vi "LEBITplc.Bob1toBunMonitor.vi"(0 "i ref in":refnum<vi>, 1 "data":i8[](array[numeric]), 2 "i attribute in":T1, 3 "index":i32, 4 "NickNames":string, 5 "error in":errorcluster, 7 "no link":bool) -> (14 "i ref out":refnum<vi>, 15 "Data":dbl[](array[numeric]), 16 "i attribute out":T1, 17 "Indexs":i32[](array[numeric]), 19 "error out":errorcluster)   [LabVIEW 2014, in "LEBITplc.lvlib"]
uses:
  LEBITplc.lvlib
  LEBITplc.i attribute.ctl
panel:
  out "No Link":bool
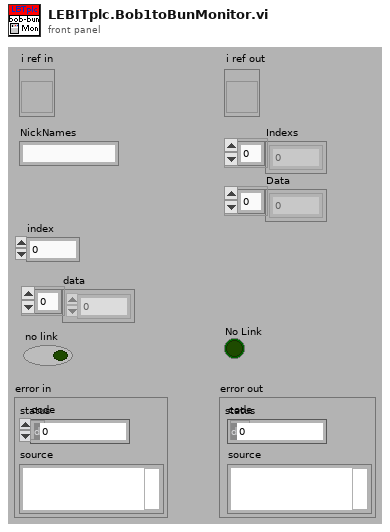
[diagram p1: front panel]
types:
  T1 = typedef "LEBITplc.lvlib/LEBITplc.i attribute.ctl" = cluster{"LLFLocation":string, "SetFileLocation":string, "nickNames":string[], "setValuePLCServiceID":i32[], "GUIServiceID":i32[], "monValuePLC":string[], "SetValueServiceID":i32[], "MonValueServiceID":i32[], "SetValue":dbl[][], "SetValueMin":dbl[], "SetValueMax":dbl[], "SetValueInfoServiceID":i32[], "GUINames":string[], "ListOfBases":string[], "Scale":dbl[], "Offset":dbl[], "setValuePLC":string[], "BaseName":string[], "ScaleServiceID":i32[], "OffsetServiceID":i32[], "AllPLCValues":string[], "CondSpecialArray":string[][], "CondSpecialIndex":i32[], "CondSpecialMonValue":dbl[], "RecentlyChanged":i32[], "SetFileLocationID":i32, "Dependent-Monitors":string[][], "LastLoadedFiles":string[], "IonGuideCalibLocation":string, "Monitor Dependent":string[], "Special":string[], "PLC?":bool[], "Start Date":string, "ListOfBasesServiceID":i32, "SETRA VISA resource":refnum<visa-resource-name>}
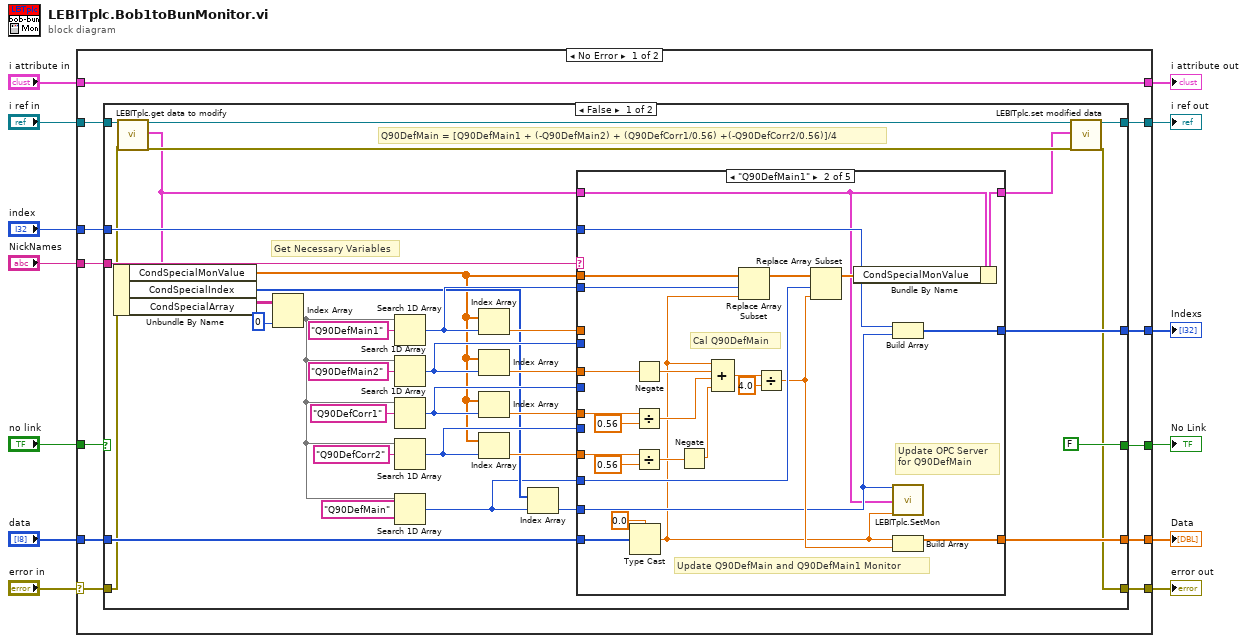
[diagram p0: block diagram]
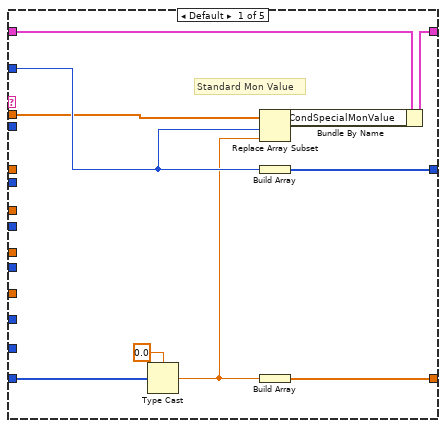
[diagram p2: hidden frame]
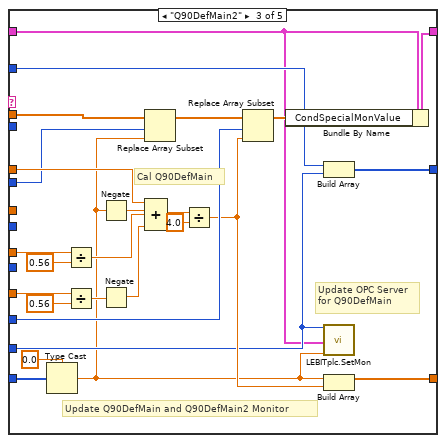
[diagram p3: hidden frame]
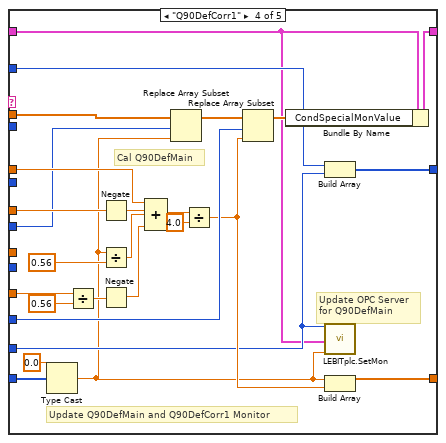
[diagram p4: hidden frame]
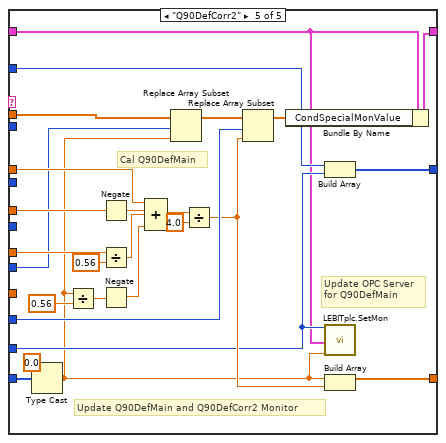
[diagram p5: hidden frame]
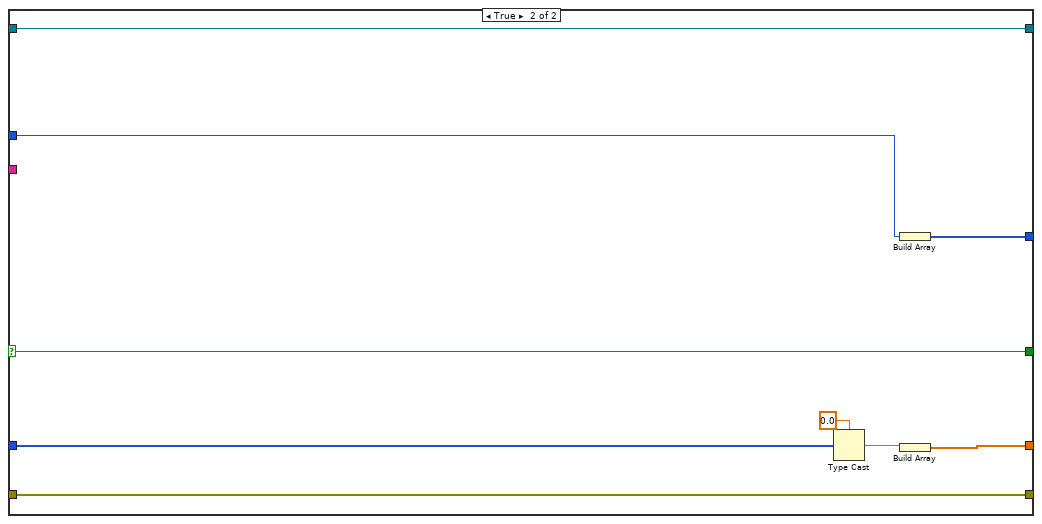
[diagram p6: hidden frame]
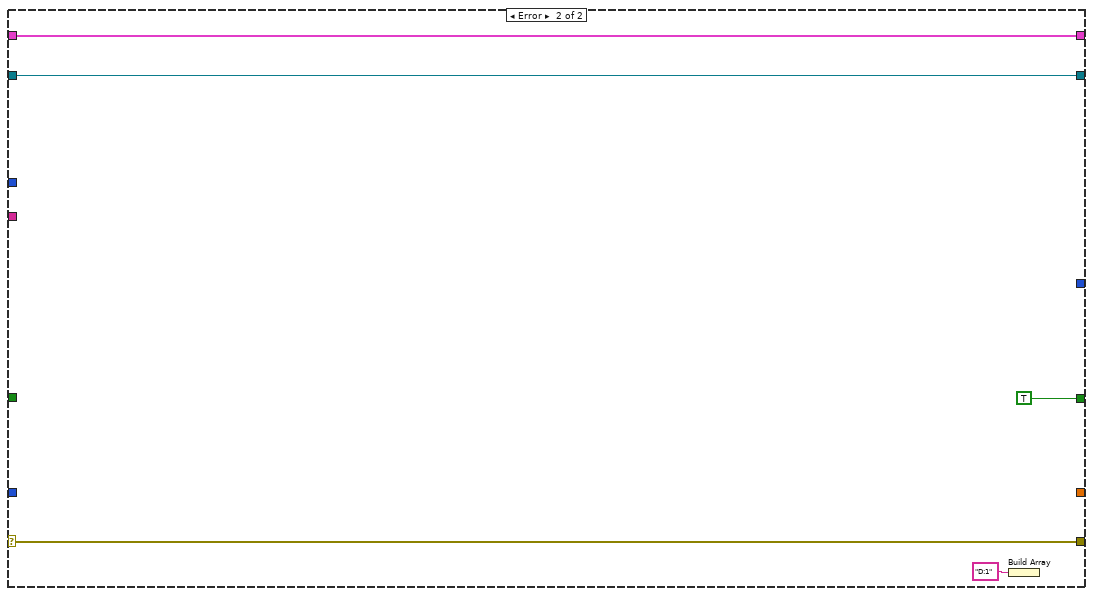
[diagram p7: hidden frame]
diagram:
  n1 = case shown="No Error" "error in" {
    selector: "error in" -> [w19 w187]
    tunnel: "NickNames" -> [w25 _]
    tunnel: [w20 w187] -> w12
    tunnel: "data" -> [w24 _]
    tunnel: "i attribute in" -> [w16 w185]
    tunnel: "i ref in" -> [w21 w186]
    tunnel: [w15 w186] -> w7
    tunnel: "index" -> [w23 _]
    tunnel: [w16 w185] -> w5
    tunnel: [w22 _] -> w4
    tunnel: "no link" -> [w18 _]
    tunnel: [w17 TRUE] -> w2
    tunnel: [w14 _] -> w1
    frame No Error {
      n2 = case shown="False" w18 {
        selector: w18 -> [_ w180]
        tunnel: w25 -> [w55 _]
        tunnel: w24 -> [w54 w175]
        tunnel: w23 -> [w48 w179]
        tunnel: [w47 w178] -> w22
        tunnel: w21 -> [w40 w182]
        tunnel: [w37 w182] -> w15
        tunnel: [w27 w181] -> w20
        tunnel: w19 -> [w26 w181]
        tunnel: [FALSE w180] -> w17
        tunnel: [w30 w174] -> w14
        frame False {
          # "Q90DefMain = [Q90DefMain1 + (-Q90DefMain2) + (Q90DefCorr1/0.56) +(-Q90DefCorr2/0.56)]/4"
          # "Get Necessary Variables"
          n3 = call "LEBITplc.get data to modify.vi"("i ref in"=w40, "error in (no error)"=w26) -> ("i ref out"=w39:refnum<vi>, "i attribute"=w28:T1, "error out"=w38:errorcluster)  [unwired: 14 in, 1 out]
          n4 = Unbundle By Name(w28) -> ("CondSpecialMonValue"=w32:dbl[], "CondSpecialIndex"=w33:i32[], "CondSpecialArray"=w59:string[][])
          n5 = Index Array(array=w59, index (col)=0 ("index (row)")) -> (element=w34:string[])  [unwired: 1 in]
          n6 = Search 1D Array(1D array=w34, element="Q90DefMain1") -> (index of element=w45:i32)  [unwired: 1 in]
          n7 = Search 1D Array(1D array=w34, element="Q90DefMain2") -> (index of element=w43:i32)  [unwired: 1 in]
          n8 = Search 1D Array(1D array=w34, element="Q90DefCorr1") -> (index of element=w44:i32)  [unwired: 1 in]
          n9 = Search 1D Array(1D array=w34, element="Q90DefCorr2") -> (index of element=w42:i32)  [unwired: 1 in]
          n10 = Search 1D Array(1D array=w34, element="Q90DefMain") -> (index of element=w29:i32)  [unwired: 1 in]
          n11 = Index Array(array=w32, index=w45) -> (element=w51:dbl)
          n12 = Index Array(array=w32, index=w43) -> (element=w50:dbl)
          n13 = Index Array(array=w32, index=w44) -> (element=w49:dbl)
          n14 = Index Array(array=w32, index=w42) -> (element=w53:dbl)
          n15 = Index Array(array=w33, index=w29) -> (element=w31:i32)
          n16 = case shown="\"Q90DefMain1\"" w55 {
            tunnel: w54 -> [w63 w94 w120 w146 w172]
            tunnel: w53 -> [_ w85 w112 w139 _]
            tunnel: w51 -> [_ _ w103 w130 w157]
            tunnel: w50 -> [_ w89 _ w128 w155]
            tunnel: w49 -> [_ w88 w115 _ w154]
            tunnel: w48 -> [w66 w78 w106 w133 w160]
            tunnel: [w69 w80 w108 w135 w162] -> w47
            tunnel: w28 -> [w67 w71 w97 w123 w149]
            tunnel: [w68 w91 w117 w143 w169] -> w36
            tunnel: w45 -> [_ w73 _ _ _]
            tunnel: w44 -> [_ _ _ w125 _]
            tunnel: w43 -> [_ _ w99 _ _]
            tunnel: w32 -> [w62 w93 w119 w145 w171]
            tunnel: w42 -> [_ _ _ _ w151]
            tunnel: w31 -> [_ w72 w98 w124 w150]
            tunnel: w29 -> [_ w79 w107 w134 w161]
            tunnel: [w61 w74 w100 w126 w152] -> w30
            frame Default {
              # "Standard Mon Value"
              n17 = Type Cast(type=0.0 ("y"), x=w63) -> (*(type *) &x=w60:dbl)
              n18 = Replace Array Subset(array=w62, new element=w60, index=w66) -> (w65:dbl[])
              n19 = Build Array(w66) -> (w69:i32[])
              n20 = Build Array(w60) -> (w61:dbl[])
              n21 = Bundle By Name(cluster=w67, "CondSpecialMonValue"=w65) -> (w68:T1)
            }
            frame "Q90DefMain1" {
              # "Update Q90DefMain and Q90DefMain1 Monitor"
              # "Update OPC Server\nfor Q90DefMain"
              # "Cal Q90DefMain"
              n22 = Type Cast(type=0.0 ("y"), x=w94) -> (*(type *) &x=w70:dbl)
              n23 = Negate(x=w89) -> (-x=w83:dbl)
              n24 = Divide(x=w88, y=0.56) -> (x/y=w82:dbl)
              n25 = Divide(x=w85, y=0.56) -> (x/y=w84:dbl)
              n26 = Negate(x=w84) -> (-x=w81:dbl)
              n27 = Compound Arithmetic op=ADD(w70, w83, w82, w81) -> (w76:dbl)
              n28 = Replace Array Subset(array=w93, new element=w70, index=w73) -> (w92:dbl[])
              n29 = Divide(x=w76, y=4.0) -> (x/y=w75:dbl)
              n30 = Replace Array Subset(array=w92, new element=w75, index=w79) -> (w90:dbl[])
              n31 = Bundle By Name(cluster=w71, "CondSpecialMonValue"=w90) -> (w91:T1)
              n32 = Build Array(w78, w72) -> (w80:i32[])
              n33 = call "LEBITplc.SetMon.vi"("index of element"=w72, "i attribute in"=w71, "Data"=w70) -> ()  [unwired: 17 in]
              n34 = Build Array(w70, w75) -> (w74:dbl[])
            }
            frame "Q90DefMain2" {
              # "Cal Q90DefMain"
              # "Update OPC Server\nfor Q90DefMain"
              # "Update Q90DefMain and Q90DefMain2 Monitor"
              n35 = Type Cast(type=0.0 ("y"), x=w120) -> (*(type *) &x=w96:dbl)
              n36 = Divide(x=w115, y=0.56) -> (x/y=w110:dbl)
              n37 = Divide(x=w112, y=0.56) -> (x/y=w111:dbl)
              n38 = Negate(x=w96) -> (-x=w102:dbl)
              n39 = Negate(x=w111) -> (-x=w109:dbl)
              n40 = Replace Array Subset(array=w119, new element=w96, index=w99) -> (w118:dbl[])
              n41 = Compound Arithmetic op=ADD(w103, w102, w110, w109) -> (w105:dbl)
              n42 = Divide(x=w105, y=4.0) -> (x/y=w101:dbl)
              n43 = Replace Array Subset(array=w118, new element=w101, index=w107) -> (w116:dbl[])
              n44 = Bundle By Name(cluster=w97, "CondSpecialMonValue"=w116) -> (w117:T1)
              n45 = Build Array(w106, w98) -> (w108:i32[])
              n46 = call "LEBITplc.SetMon.vi"("index of element"=w98, "i attribute in"=w97, "Data"=w96) -> ()  [unwired: 17 in]
              n47 = Build Array(w96, w101) -> (w100:dbl[])
            }
            frame "Q90DefCorr1" {
              # "Update OPC Server\nfor Q90DefMain"
              # "Cal Q90DefMain"
              # "Update Q90DefMain and Q90DefCorr1 Monitor"
              n48 = Type Cast(type=0.0 ("y"), x=w146) -> (*(type *) &x=w122:dbl)
              n49 = Divide(x=w139, y=0.56) -> (x/y=w138:dbl)
              n50 = Negate(x=w128) -> (-x=w129:dbl)
              n51 = Divide(x=w122, y=0.56) -> (x/y=w137:dbl)
              n52 = Negate(x=w138) -> (-x=w136:dbl)
              n53 = Compound Arithmetic op=ADD(w130, w129, w137, w136) -> (w132:dbl)
              n54 = Replace Array Subset(array=w145, new element=w122, index=w125) -> (w144:dbl[])
              n55 = Divide(x=w132, y=4.0) -> (x/y=w127:dbl)
              n56 = Replace Array Subset(array=w144, new element=w127, index=w134) -> (w142:dbl[])
              n57 = Bundle By Name(cluster=w123, "CondSpecialMonValue"=w142) -> (w143:T1)
              n58 = Build Array(w133, w124) -> (w135:i32[])
              n59 = call "LEBITplc.SetMon.vi"("index of element"=w124, "i attribute in"=w123, "Data"=w122) -> ()  [unwired: 17 in]
              n60 = Build Array(w122, w127) -> (w126:dbl[])
            }
            frame "Q90DefCorr2" {
              # "Update Q90DefMain and Q90DefCorr2 Monitor"
              # "Update OPC Server\nfor Q90DefMain"
              # "Cal Q90DefMain"
              n61 = Type Cast(type=0.0 ("y"), x=w172) -> (*(type *) &x=w148:dbl)
              n62 = Divide(x=w148, y=0.56) -> (x/y=w165:dbl)
              n63 = Negate(x=w155) -> (-x=w156:dbl)
              n64 = Divide(x=w154, y=0.56) -> (x/y=w164:dbl)
              n65 = Negate(x=w165) -> (-x=w163:dbl)
              n66 = Compound Arithmetic op=ADD(w157, w156, w164, w163) -> (w159:dbl)
              n67 = Replace Array Subset(array=w171, new element=w148, index=w151) -> (w170:dbl[])
              n68 = Divide(x=w159, y=4.0) -> (x/y=w153:dbl)
              n69 = Replace Array Subset(array=w170, new element=w153, index=w161) -> (w168:dbl[])
              n70 = Bundle By Name(cluster=w149, "CondSpecialMonValue"=w168) -> (w169:T1)
              n71 = Build Array(w160, w150) -> (w162:i32[])
              n72 = call "LEBITplc.SetMon.vi"("index of element"=w150, "i attribute in"=w149, "Data"=w148) -> ()  [unwired: 17 in]
              n73 = Build Array(w148, w153) -> (w152:dbl[])
            }
          }
          n74 = call "LEBITplc.set modified data.vi"("i ref in"=w39, "i attribute"=w36, "error in (no error)"=w38) -> ("i ref out"=w37:refnum<vi>, "error out"=w27:errorcluster)  [unwired: 15 in]
        }
        frame True {
          n75 = Type Cast(type=0.0, x=w175) -> (*(type *) &x=w176:dbl)
          n76 = Build Array(w179) -> (w178:i32[])
          n77 = Build Array(w176) -> (w174:dbl[])
        }
      }
    }
    frame Error {
      n78 = Build Array("D:1" ("element")) -> ()  [unwired: 1 out]
    }
  }
  "error out" <- w12
  "i ref out" <- w7
  "i attribute out" <- w5
  "Indexs" <- w4
  "No Link" <- w2
  "Data" <- w1
